vi "Is square occupied.vi"(8 "error in (no error)":errorcluster, 10 "Square":T1={"File"=enum."a", "Rank"=enum."4"}, 11 "Board in":refnum<class "Board.lvclass">) -> (0 "error out":errorcluster, 2 "Occupied":bool, 3 "Board out":refnum<class "Board.lvclass">)   [LabVIEW 2016, in "Chesslib.lvlib" / "Board.lvclass"]
uses:
  Board.lvclass
  typedef/Square.ctl
  typedef/File.ctl
  typedef/Rank.ctl
  Board.lvclass/Board.ctl
  Chesslib.lvlib
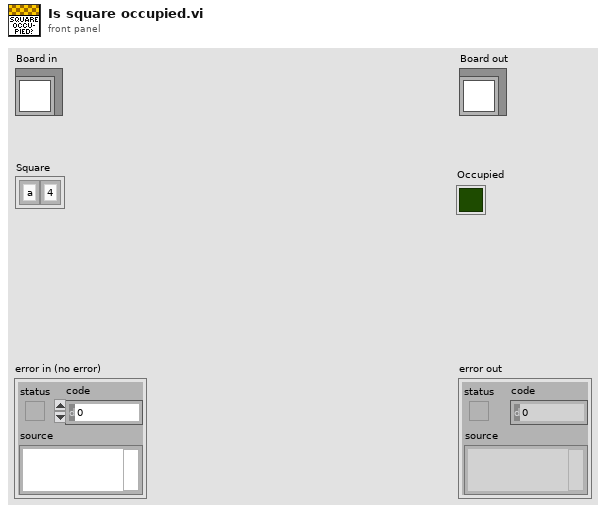
[diagram p1: front panel]
types:
  T1 = typedef "Chesslib.lvlib/Square.ctl" = cluster{"File":T2, "Rank":T3}
  T2 = typedef "Chesslib.lvlib/File.ctl" = enum8{"a", "b", "c", "d", "e", "f", "g", "h"}
  T3 = typedef "Chesslib.lvlib/Rank.ctl" = enum8{"1", "2", "3", "4", "5", "6", "7", "8"}
  T4 = typedef "Chesslib.lvlib/Board.lvclass/Square content.ctl" = cluster{"Occupied":bool, "Piece":refnum<class "Piece.lvclass">}
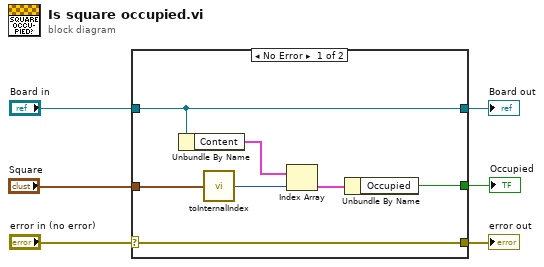
[diagram p0: block diagram]
diagram:
  n1 = case shown="No Error" "error in (no error)" {
    selector: "error in (no error)" -> [w13 w15]
    tunnel: [w13 w15] -> w5
    tunnel: [w12 w14] -> w3
    tunnel: "Board in" -> [w12 w14]
    tunnel: "Square" -> [w11 _]
    tunnel: [w7 _] -> w1
    frame No Error {
      n2 = Unbundle By Name(w12) -> ("Content"=w10:T4[])
      n3 = call "toInternalIndex.vi"("Square"=w11) -> ("Internal index"=w9:i32)
      n4 = Index Array(array=w10, index=w9) -> (element=w8:T4)
      n5 = Unbundle By Name(w8) -> ("Occupied"=w7:bool)
    }
    frame Error {
    }
  }
  "error out" <- w5
  "Board out" <- w3
  "Occupied" <- w1
